vi "Invoke RT VI.vi"(6 "Run Time":u32, 7 "error in (no error)":errorcluster, 9 "configuration file path":path, 10 "target alias":string, 11 "reference":refnum<vi>) -> (0 "error out":errorcluster, 3 "reference out":refnum<vi>, 4 "invoked VI error out":errorcluster)   [LabVIEW 2014]
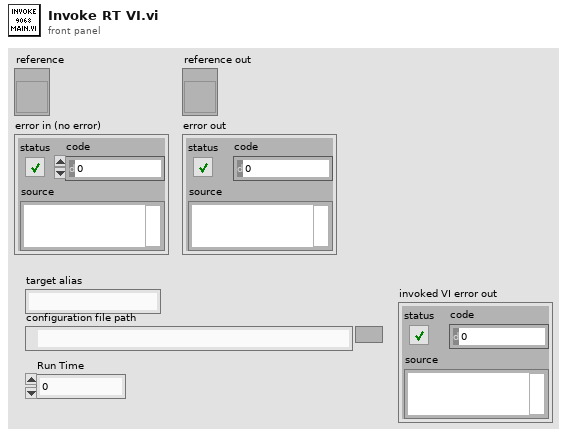
[diagram p1: front panel]
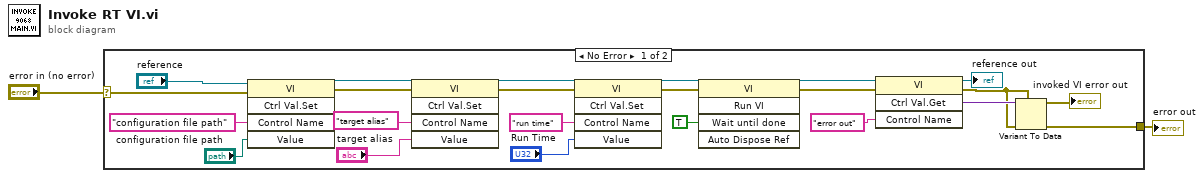
[diagram p0: block diagram]
diagram:
  n1 = case shown="No Error" "error in (no error)" {
    selector: "error in (no error)" -> [w3 w26]
    tunnel: [w8 w26] -> w2
    frame No Error {
      n2 = invoke class="VI" method="Ctrl Val.Set"(reference="reference", error in=w3, "Control Name"="configuration file path", "Value"="configuration file path") -> (reference out=w6:refnum<vi>, error out=w14:errorcluster)  [unwired: 1 in, 3 out]
      n3 = invoke class="VI" method="Ctrl Val.Set"(reference=w6, error in=w14, "Control Name"="target alias", "Value"="target alias") -> (reference out=w17:refnum<vi>, error out=w16:errorcluster)  [unwired: 1 in, 3 out]
      n4 = invoke class="VI" method="Ctrl Val.Set"(reference=w17, error in=w16, "Control Name"="run time", "Value"="Run Time") -> (reference out=w19:refnum<vi>, error out=w20:errorcluster)  [unwired: 1 in, 3 out]
      n5 = invoke class="VI" method="Run VI"(reference=w19, error in=w20, "Wait until done"=TRUE ("Wait Until Done")) -> (reference out=w21:refnum<vi>, error out=w24:errorcluster)  [unwired: 2 in, 3 out]
      n6 = invoke class="VI" method="Ctrl Val.Get"(reference=w21, error in=w24, "Control Name"="error out") -> (reference out=→"reference out":refnum<vi>, error out=w7:errorcluster, "Get Control Value Variant"=w23:variant)  [unwired: 1 in, 1 out]
      n7 = Variant To Data(error in=w7, type=w7, Variant=w23) -> (data=→"invoked VI error out":errorcluster, error out=w8:errorcluster)
    }
    frame Error {
    }
  }
  "error out" <- w2
